vi "3_ImClass(Deploy)(File).vi"() -> ()   [LabVIEW 2020]
doc: "This example demonstrates the process of loading pretrained model for objects detection and running for inference/prediction.\nRequirements: 1. Deep Learning Toolkit for LabVIEW (v3.0 and above).\n 2. NI Vision Development Module.\n 3. Trained model generated during training."
uses:
  <vilib>/Ngene/Deep Learning Toolkit/Toolkit/NN_Network/Controls/NN_Device.ctl
  <vilib>/Ngene/Deep Learning Toolkit/Toolkit/NN_Data/API/NN_Dims(C,H,W).ctl
  <vilib>/Ngene/Deep Learning Toolkit/Toolkit/NN_Network/Controls/NN_Save_Before_Destroy_Options.ctl
  <vilib>/Ngene/Deep Learning Toolkit/Toolkit/NN_Network/API/NN_Set_Input/3D/NN_Set_Input(3D_SGL_idx).vi
  <vilib>/Ngene/Deep Learning Toolkit/Toolkit/NN_Data/subVIs/Get_Data_Vals/2D/NN_Data_Get_ValByRef(2D_SGL_idx).vi
  <vilib>/Ngene/Deep Learning Toolkit/Toolkit/Deep_Learning_Toolkit_by_Ngene.lvlib
panel:
  out "Dims_In":T1={"C"=3, "H"=32, "W"=32}
  out "Labels":string[](array[string])=["airplane", "automobile", "bird", "cat", "deer", "dog", "frog", "horse", "ship", "truck"]
  out "Predictions":sgl[](array[slide])=[0.07841631, 0.009722123, 0.4336321, 0.036632217, 0.019995471, 0.019788245, 0.08266291, 0.014530446, 0.17630611, 0.12831411] scale=0.0..1.0
  out "Inference Time":dbl=0.014362300000357209 format="%#_5p"
  out "Sample Path":path=path "D:/DNN/CIFAR-10_Images/Test/bird/bird_01852.bmp"
  in  "Select Sample":i32=2179 min=0 max=9999 step=1
  in  "Dataset Path (Images)":path=path "D:/DNN/CIFAR-10_Images/Test"
  in  "NN_Device":T2
  out "FPS":dbl=69.62673109287013 format="%#_4f"
  out "Input Image":T3(plugin-control)
  in  "Stop":bool
  in  "Model Weights":path=path "D:/working/ImClass/ImClass_weights_25_04_18__18_42_33.bin"
  in  "Model Topology (CFG)":path=path "D:/working/ImClass/ImClass_net_cfg_25_04_18__18_42_33.cfg"
  # "Overview: This example demonstrates the process of loading a pretrained model for image classification and running inference/prediction.\nRequirements:\nDeep Learning Toolkit for LabVIEW\nNI Vision Development Module.\nTrained model generated during training.\nInstructions:\n1. Provide the \"Model Topology (CFG)\" and \"Model Weights\" generated after training.\n2. Set the \"Dataset Path (Images)\" to the folder containing the test images.\n3. Run the VI.\n4. Use \"Select Sample\" to choose different image samples from the dataset.\n5. Press \"Stop\" to end the VI.\nMore Examples:  https://github.com/ngenehub/deepltk_examples"
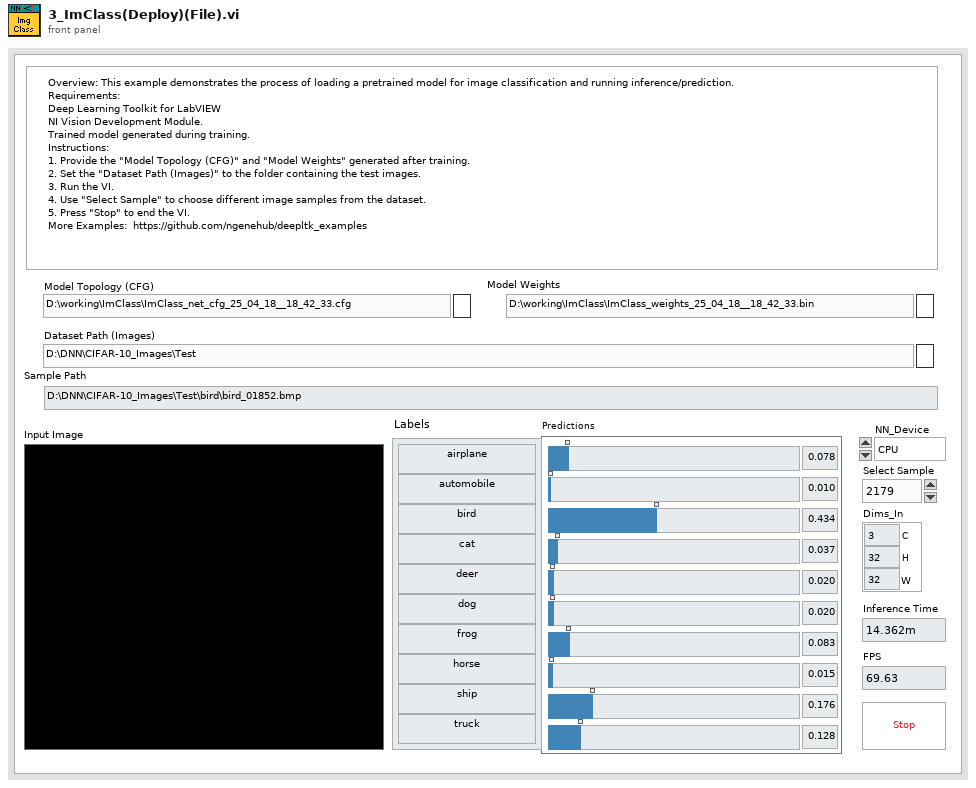
[diagram p1: front panel]
types:
  T1 = typedef "Deep_Learning_Toolkit_by_Ngene.lvlib/NN_Dims(C,H,W).ctl" = cluster{"C":i32, "H":i32, "W":i32}
  T2 = typedef "Deep_Learning_Toolkit_by_Ngene.lvlib/NN_Device.ctl" = enum16{"CPU", "GPU"}
  T3 = typedef "IMAQ Image.ctl" = refnum<image>
  T4 = typedef "Deep_Learning_Toolkit_by_Ngene.lvlib/NN_Save_Before_Destroy_Options.ctl" = cluster{"CFG?":bool, "Weights?":bool, "Render?":bool}
  T5 = typedef "Deep_Learning_Toolkit_by_Ngene.lvlib/NN_Config_Params.ctl" = cluster{"Name":string, "mBatch":i32, "NN_Train_Params":T6, "LR_Decay_Policy":T9, "Labels":string[], "Loss":T11}
  T6 = typedef "Deep_Learning_Toolkit_by_Ngene.lvlib/NN_Train_Params.ctl" = cluster{"Optimizer":T7, "Beta_1":sgl, "Beta_2":sgl, "Weight Decay(L1)":sgl, "Weight Decay(L2)":sgl, "Data_Sampling":T8}
  T7 = typedef "Deep_Learning_Toolkit_by_Ngene.lvlib/NN_Train_Optimizer.ctl" = enum16{"SGD", "Adam", "Adagrad", "Adadelta", "RMSProp", "Nesterov"}
  T8 = typedef "Deep_Learning_Toolkit_by_Ngene.lvlib/NN_Train_Data_Sampling.ctl" = enum16{"Random", "Sequential"}
  T9 = typedef "Deep_Learning_Toolkit_by_Ngene.lvlib/NN_LR_Policy_Cfg.ctl" = cluster{"Policy_Type":T10, "LR0":dbl, "k":sgl, "WarmUp_Policy":enum16{"Step", "Ramp"}, "WarmUp_Iter":i32, "WarmUp_Ratio":sgl}
  T10 = typedef "Deep_Learning_Toolkit_by_Ngene.lvlib/NN_LR_Policy_Type.ctl" = enum16{"Manual", "Step", "Exp", "1/t"}
  T11 = typedef "Deep_Learning_Toolkit_by_Ngene.lvlib/NN_Loss_Config_Params.ctl" = cluster{"Loss_Type":T12, "Loss_Conf_Params":variant}
  T12 = typedef "Deep_Learning_Toolkit_by_Ngene.lvlib/NN_Loss_Type.ctl" = enum16{"None", "MSE", "CrossEntropy", "YOLO_v2", "YOLO_v4"}
  T13 = typedef "Deep_Learning_Toolkit_by_Ngene.lvlib/NN_Layer_Config_Params.ctl" = cluster{"Layer_Type":T14, "Layer_Conf_Params":variant, "Input Layers":string[]}
  T14 = typedef "Deep_Learning_Toolkit_by_Ngene.lvlib/NN_Layer_Type.ctl" = enum16{"Input1D", "Input3D", "Conv1D", "Conv2D", "Conv2D_Adv", "MaxPool", "AvgPool", "UpSample", "DropOut3D", "ShortCut", "Concat", "SoftMax3D", "FC", "DropOut", "Softmax", "Flatten", "YOLO_v2", "YOLO_v4", "Activation", "BatchNormalization", "Unsupported"}
  T15 = typedef "Deep_Learning_Toolkit_by_Ngene.lvlib/NN.ctl" = cluster{"Name":string, "No of Layers":i32, "mBatch":i32, "Layers":T16[], "Dimty":T17, "Dims_In":T1, "Dims_Out":T1, "Working_Dir":path, "Train?":bool, "Train_Params":T6, "LR_Update_Policy":T9, "Session Data":T18, "Ground_truth":T19, "NNg_hdls":T20, "NN_Device":T2, "GPU Id":i32, "Labels":string[], "Receptive Field":T21[], "Loss_Type":T12, "Loss_Cfg_Prms":variant, "NNG_WS":T22}
  T16 = typedef "Deep_Learning_Toolkit_by_Ngene.lvlib/NN_Layer_ref.ctl" = refnum<data-value>
  T17 = typedef "Deep_Learning_Toolkit_by_Ngene.lvlib/NN_In_Out_Dim-ty.ctl" = enum8{"In1D_Out1D", "In3D_Out1D", "In3D_Out3D", "In3D_OutBBox"}
  T18 = typedef "Deep_Learning_Toolkit_by_Ngene.lvlib/NN_Train_Session_Data.ctl" = cluster{"Epochs":sgl, "Tot_Iter":i32, "LR":sgl, "LR_iter":i32}
  T19 = typedef "Deep_Learning_Toolkit_by_Ngene.lvlib/NN_Ground_truth.ctl" = cluster{"Y":variant}
  T20 = typedef "Deep_Learning_Toolkit_by_Ngene.lvlib/nng_cuda_handles.ctl" = cluster{"cudnn":u64, "cublas":u64, "stream":u64, "curand":u64}
  T21 = typedef "Deep_Learning_Toolkit_by_Ngene.lvlib/NN_Dims(V,H).ctl" = cluster{"V":i32, "H":i32}
  T22 = typedef "Deep_Learning_Toolkit_by_Ngene.lvlib/NNG_WS.ctl" = cluster{"NNG_WS_Mem":T23, "Max_WS_Size":i64}
  T23 = typedef "Deep_Learning_Toolkit_by_Ngene.lvlib/NNg_WS_Mem_DVR.ctl" = refnum<data-value>
  T24 = typedef "Deep_Learning_Toolkit_by_Ngene.lvlib/NN_Layer.ctl" = cluster{"Name":string, "Layer_Data":variant, "Layer_Type":T14, "Dims_In":T1, "Layers_In":variant, "Dims_Out":T1, "Layers_Out":variant, "Metrics":T25, "GPU_Data":variant, "mBatch":i32, "NN_Device":T2, "NNg_hdls":T20, "Train?":bool, "Dimty":T26, "RecptField":T27}
  T25 = typedef "Deep_Learning_Toolkit_by_Ngene.lvlib/NN_Layer_Metrics.ctl" = cluster{"Data":dbl, "Params":dbl, "Ops":dbl}
  T26 = typedef "Deep_Learning_Toolkit_by_Ngene.lvlib/NN_Layer_Dimty.ctl" = enum16{"1D", "3D"}
  T27 = typedef "Deep_Learning_Toolkit_by_Ngene.lvlib/NN_Layer_RF_State.ctl" = cluster{"Dims":T21, "J":T21}
  T28 = typedef "Deep_Learning_Toolkit_by_Ngene.lvlib/NN_Data_ref(2D_SGL).ctl" = refnum<data-value>
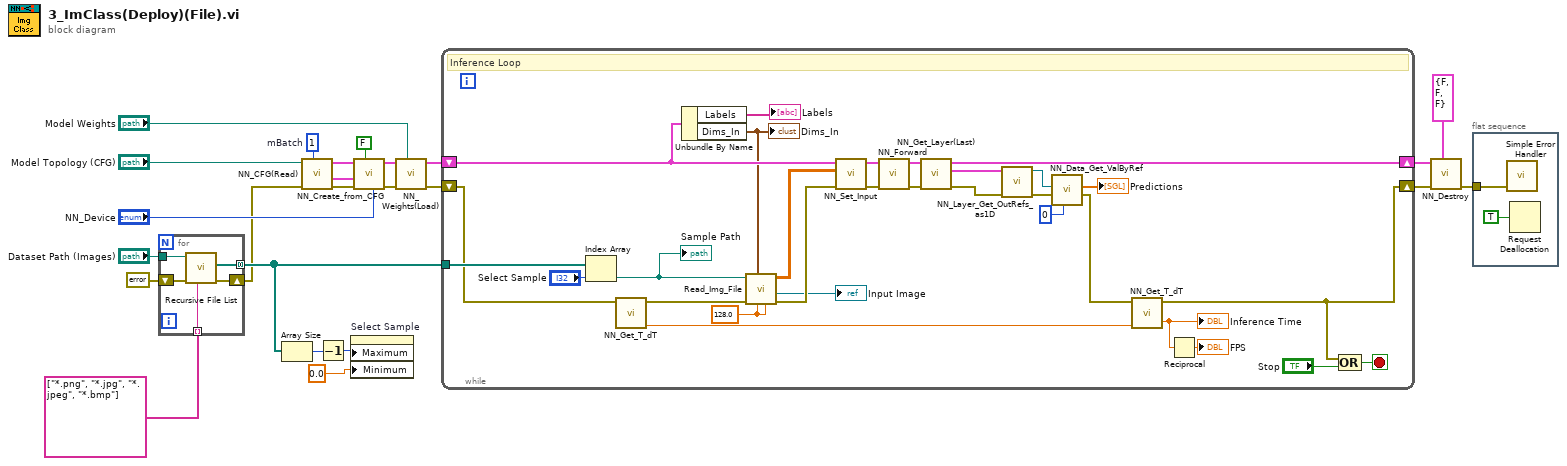
[diagram p0: block diagram]
diagram:
  w10 = 1  # mBatch
  n1 = for {
    tunnel: "Dataset Path (Images)" -> [w29]
    tunnel: string[] ["*.png", "*.jpg", "*.jpeg", "*.bmp"] ("pattern") -> [w28] mode=indexing
    tunnel: [w27] -> w6 mode=concatenating
    shift-right: [w25] -> w3
    shift-left: errorcluster {"status"=FALSE, "code"=0, "source"=""} ("error out") -> [w26]
    n2 = call <vilib>:"Recursive File List.vi"("pattern"=w28, "error in (no error)"=w26, "Folder Path"=w29) -> ("error out"=w25:errorcluster, "All Files in Dir"=w27:path[])  [unwired: 4 in, 3 out]
  }
  n3 = Array Size(array=w6) -> (size(s)=w7:i32)
  n4 = call <vilib>:"NN_CFG(Read).vi"("mBatch"=w10, "error in (no error)"=w3, "CFG file path"="Model Topology (CFG)") -> ("error out"=w22:errorcluster, "Net_Cfg"=w9:T5, "Layer_Cfg"=w23:T13[])  [unwired: 6 in]
  n5 = Decrement(x=w7) -> (x-1=w5:i32)
  n6 = property on="Select Sample" class="DigNum (strict)"("Maximum"=w5, "Minimum"=0.0 ("Data Entry Limits:Minimum")) -> ()  [unwired: 2 in, 2 out]
  n7 = call <vilib>:"NN_Create_from_CFG.vi"("NN_Device"="NN_Device", "Train? (false)"=FALSE ("Train?"), "error in (no error)"=w22, "Net_Cfg"=w9, "Layer_Cfg"=w23) -> ("error out"=w21:errorcluster, "NN out"=w19:T15)  [unwired: 5 in]
  n8 = call <vilib>:"NN_Weights(Load).vi"("Weight File Path"="Model Weights", "error in (no error)"=w21, "NN in"=w19) -> ("error out"=w1:errorcluster, "NN out"=w4:T15)  [unwired: 7 in]
  n9 = while {
    shift-right: [w43] -> w18
    shift-left: w4 -> [w37]
    tunnel: w6 -> [w57]
    shift-right: [w50] -> w12
    shift-left: w1 -> [w55]
    stop <- w58 stop-if-true
    w32 = sgl 128.0 ("Shift")
    # "Inference Loop"
    n10 = Index Array(array=w57, index="Select Sample") -> (element=w38:path)
    "Sample Path" <- w38
    n11 = call <vilib>:"NN_Get_T_dT.vi"("error in (no error)"=w55) -> ("T_out"=w47:dbl, "error out"=w34:errorcluster)  [unwired: 6 in, 1 out]
    n12 = Unbundle By Name(w37) -> ("Labels"=→"Labels":string[], "Dims_In"=w36:T1)
    "Dims_In" <- w36
    n13 = call "Read_Img_File.vi"("Divider"=w32, "Shift"=w32, "Dims(C,H,W)"=w36, "error in (no error)"=w34, "Path"=w38) -> ("error out"=w33:errorcluster, "ReadDsInput"=→"Input Image":T3, "Data"=w35:sgl[][][])  [unwired: 3 in, 1 out]
    n14 = call-poly <vilib>:"NN_Set_Input.vi"("error in (no error)"=w33, "Data_In(3D_SGL)"=w35, "NN in"=w37) -> ("error out"=w51:errorcluster, "NN out"=w52:T15)  [unwired: 7 in]
    n15 = call <vilib>:"NN_Forward.vi"("error in (no error)"=w51, "NN in"=w52) -> ("error out"=w53:errorcluster, "NN out"=w54:T15)  [unwired: 6 in, 2 out]
    n16 = call <vilib>:"NN_Get_Layer(Last).vi"("error in (no error)"=w53, "NN in"=w54) -> ("error out"=w44:errorcluster, "Last_Layer"=w45:T24, "NN out"=w43:T15)  [unwired: 6 in, 1 out]
    n17 = call <vilib>:"NN_Layer_Get_OutRefs_as1D.vi"("error in (no error)"=w44, "Layer"=w45) -> ("error out"=w41:errorcluster, "Out"=w46:T28)  [unwired: 7 in, 1 out]
    n18 = call-poly <vilib>:"NN_Data_Get_ValByRef.vi"("index (row)"=0, "error in (no error)"=w41, "DVR(2D_SGL)"=w46) -> ("error out"=w40:errorcluster, "Value(1D_SGL)"=→"Predictions":sgl[])  [unwired: 5 in]
    n19 = call <vilib>:"NN_Get_T_dT.vi"("T_in"=w47, "error in (no error)"=w40) -> ("error out"=w50:errorcluster, "dT"=w49:dbl)  [unwired: 5 in, 1 out]
    "Inference Time" <- w49
    n20 = Reciprocal(x=w49) -> (1/x=→"FPS":dbl)
    n21 = Compound Arithmetic op=OR(w50, "Stop") -> (w58:bool)
  }
  n22 = call <vilib>:"NN_Destroy.vi"("Save (T, T, T)"=T4 {"CFG?"=FALSE, "Weights?"=FALSE, "Render?"=FALSE} ("Save_Config"), "error in (no error)"=w12, "NN in"=w18) -> ("error out"=w11:errorcluster)  [unwired: 7 in, 1 out]
  n23 = flat-sequence {
    tunnel: w11 -> [w60]
    frame #0 {
      n24 = call <vilib>:"Simple Error Handler.vi"("error in (no error)"=w60) -> ()  [unwired: 4 in, 5 out]
      n25 = Request Deallocation(TRUE ("flag")) -> ()
    }
  }
